vi "_RT_CtrlLoop_D999_Setting_Cmd.vi"(7 "CmdParam":T1={"Cmd"=enum."Init", "Variant"=variant}, 8 "error in (no error)":errorcluster, 10 "VISA resource In":refnum<visa-resource-name>, 11 "headcmd in":string) -> (0 "error out":errorcluster, 1 "valid":bool, 2 "VISA resource Out":refnum<visa-resource-name>, 3 "headcmd out":string, 4 "Response Str":string)   [LabVIEW 2018]
uses:
  PublicSubVI/Ctl/_ctl_RT_D999_Settings.ctl
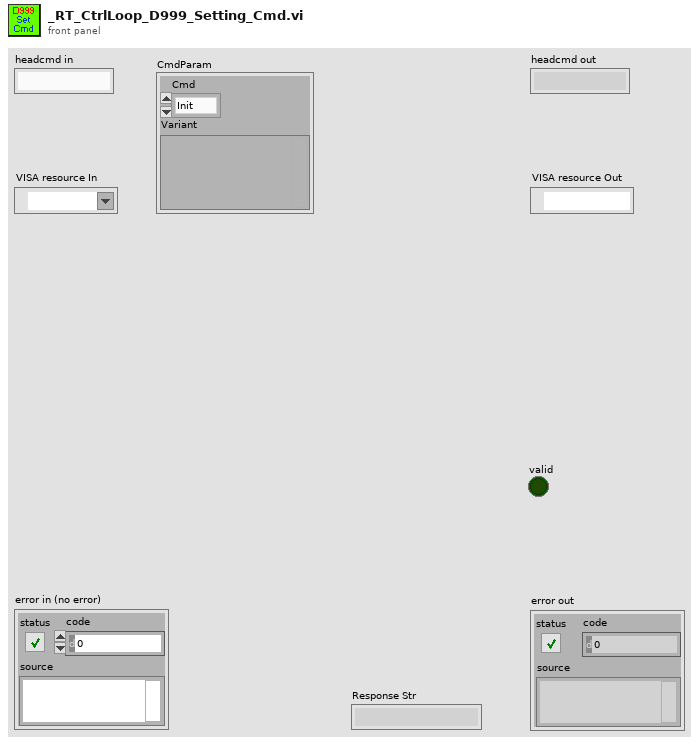
[diagram p1: front panel]
types:
  T1 = typedef "_ctl_RT_D999_Settings.ctl" = cluster{"Cmd":enum16{"None", "Init", "Write", "WriteAll", "Read", "ReadAll", "SetEnable", "SetParam", "ReadAO", "ReadSwitch", "ReportID"}, "Variant":variant}
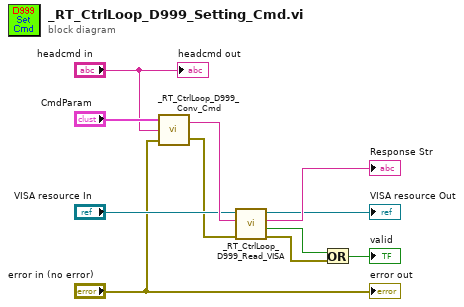
[diagram p0: block diagram]
diagram:
  n1 = call "_RT_CtrlLoop_D999_Conv_Cmd.vi"("error in (no error)"="error in (no error)", "Head+Addr+Seg"="headcmd in", "CmdParam"="CmdParam") -> ("error out"=w7:errorcluster, "Cmd_String"=w11:string)
  n2 = call "_RT_CtrlLoop_D999_Read_VISA.vi"("error in (no error)"=w7, "Comm Str"=w11, "VISA resource In"="VISA resource In") -> ("error out"=w1:errorcluster, "Is Exist?"=w2:bool, "Response Str"=→"Response Str":string, "VISA resource Out"=→"VISA resource Out":refnum<visa-resource-name>)  [unwired: 5 in]
  n3 = Or(x=w2, y=w1) -> (x .or. y?=→"valid":bool)
  "error out" <- "error in (no error)"
  "headcmd out" <- "headcmd in"
